vi "DB - Update [Table] Set [ColNames] equ Data.vi"(10 "<Data> (0xFFFE autodetect)":string[](array[string]), 11 "[ColumnNames]":string[](array[string])) -> (3 "<Values>":string)   [LabVIEW 2020]
panel:
  # "[abc]\n[def]\n[hij]"
  # "123\n456\nunicode"
  # "[abc] = '123'  ,[def] = '456' , [hij] = CONVERT(varbinary(max),'0xFFFE343536',1)"
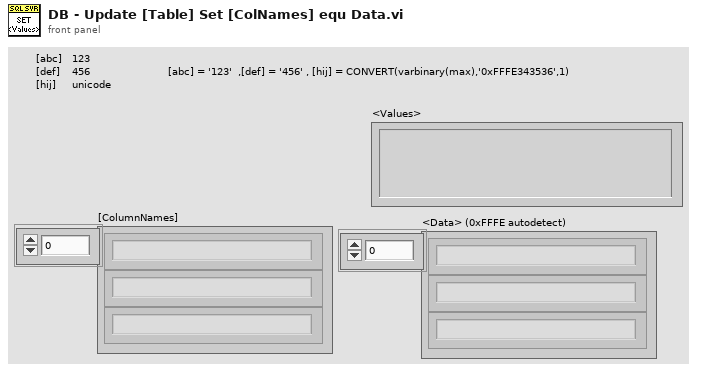
[diagram p1: front panel]
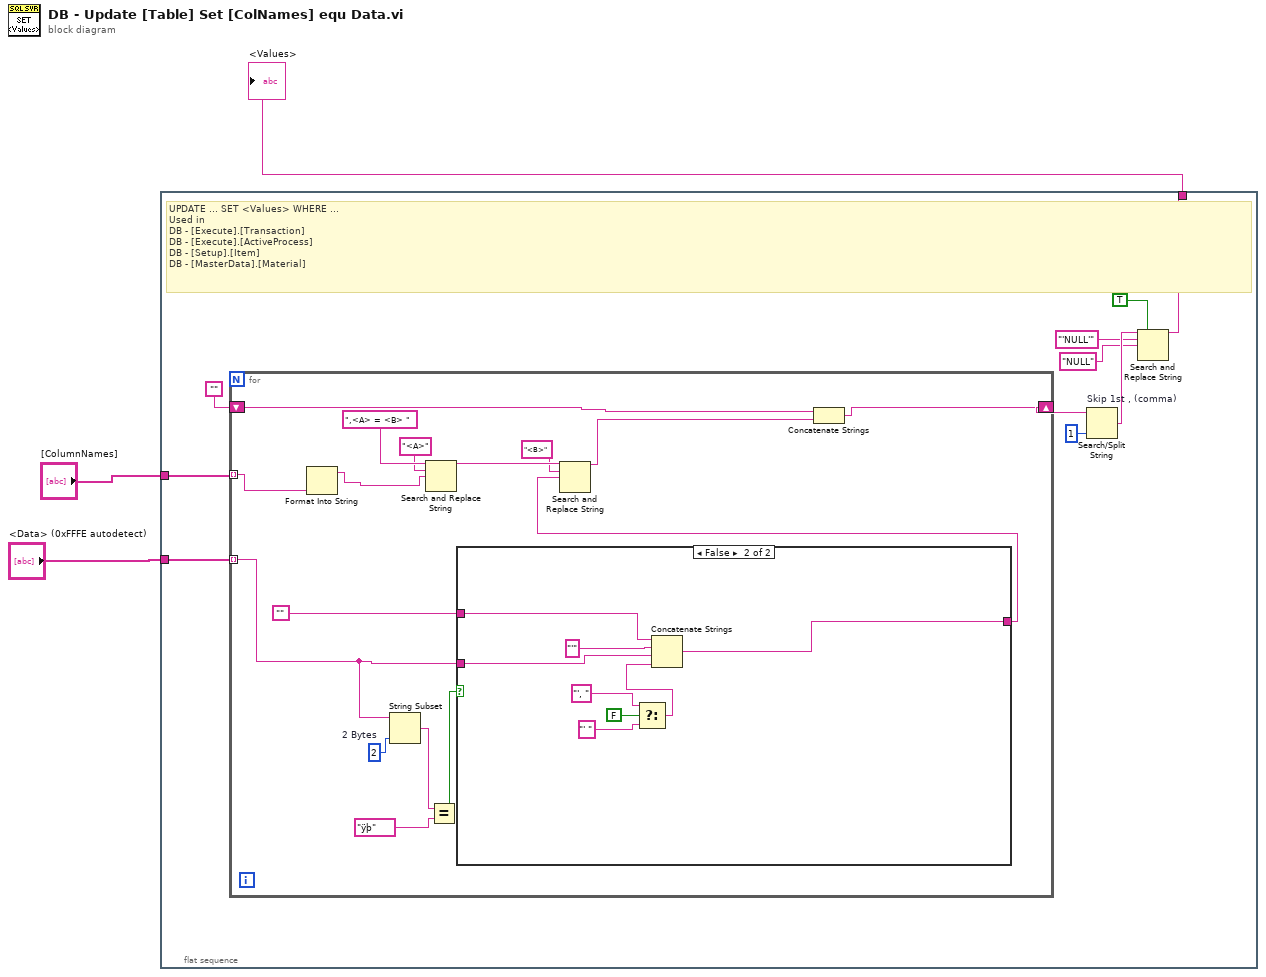
[diagram p0: block diagram]
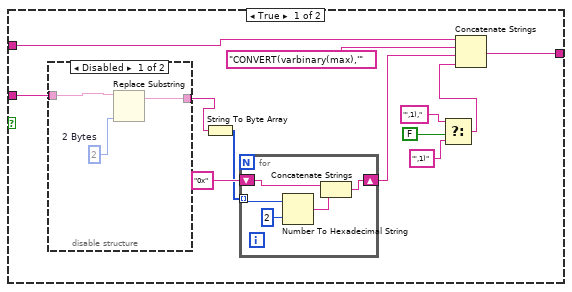
[diagram p2: hidden frame]
diagram:
  n1 = flat-sequence {
    tunnel: [w6] -> w2
    tunnel: "[ColumnNames]" -> [w5]
    tunnel: "<Data> (0xFFFE autodetect)" -> [w4]
    frame #0 {
      # "UPDATE ... SET <Values> WHERE ...\nUsed in \nDB - [Execute].[Transaction]\nDB - [Execute].[ActiveProcess]\nDB - [Setup].[Item]\nDB - [MasterData].[Material]"
      n2 = for {
        tunnel: w5 -> [w22] mode=indexing
        tunnel: w4 -> [w15] mode=indexing
        shift-right: [w23] -> w11
        shift-left: "" -> [w25]
        w20 = 2  # 2 Bytes
        n3 = Format Into String(w22) -> (resulting string=w21:string)  [unwired: 3 in, 1 out]
        n4 = String Subset(string=w15, length (rest)=w20) -> (substring=w19:string)  [unwired: 1 in]
        n5 = Search and Replace String(input string=",<A> = <B> ", search string="<A>", replace string=w21) -> (result string=w27:string)  [unwired: 5 in, 3 out]
        n6 = Equal?(x=w19, y="ÿþ" ("search string")) -> (x = y?=w17:bool)
        n7 = case shown="False" w17 {
          tunnel: "" -> [w36 w58]
          tunnel: [w34 w57] -> w14
          tunnel: w15 -> [w41 w55]
          frame True {
            n8 = disable-structure shown="Disabled" {
              disable-tunnel: w41 -> [w44 w45]
              disable-tunnel: [w42 w45] -> w37
              frame Disabled {
                w43 = 2  # 2 Bytes
                n9 = Replace Substring(2:w43, 5:w44) -> (1:w42:string)  [unwired: 2 in, 1 out]
              }
              frame Enabled {
              }
            }
            n10 = String To Byte Array(string=w37) -> (unsigned byte array=w38:u8[])
            n11 = for {
              tunnel: w38 -> [w50] mode=indexing
              shift-right: [w48] -> w35
              shift-left: "0x" -> [w47]
              n12 = Number To Hexadecimal String(1:i16 2 ("width (-)"), 2:w50) -> (0:w49:string)
              n13 = Concatenate Strings(w47, w49) -> (w48:string)
            }
            n14 = Select(t="',1)," ("string"), s=FALSE, f="',1)" ("string")) -> (s? t:f=w30:string)
            n15 = Concatenate Strings(w36, "CONVERT(varbinary(max),'" ("string"), w35, w30) -> (w34:string)
          }
          frame False {
            n16 = Select(t="', ", s=FALSE, f="' ") -> (s? t:f=w52:string)
            n17 = Concatenate Strings(w58, "'", w55, w52) -> (w57:string)
          }
        }
        n18 = Search and Replace String(input string=w27, search string="<B>", replace string=w14) -> (result string=w24:string)  [unwired: 5 in, 3 out]
        n19 = Concatenate Strings(w25, w24) -> (w23:string)
      }
      n20 = Search/Split String "Skip 1st , (comma)"(string=w11, offset (0)=1) -> (match + rest of string=w10:string)  [unwired: 1 in, 2 out]
      n21 = Search and Replace String(replace all?=TRUE ("replace all? (F)"), input string=w10, search string="'NULL'", replace string="NULL" ("replace string (\"\")")) -> (result string=w6:string)  [unwired: 4 in, 3 out]
    }
  }
  "<Values>" <- w2
